vi "Read Frequency.vi"(8 "error in (no error)":errorcluster, 11 "Set Frequency Message in":refnum<class "Set Frequency Message.lvclass">) -> (0 "error out":errorcluster, 2 "Frequency":dbl, 3 "Set Frequency Message out":refnum<class "Set Frequency Message.lvclass">)   [LabVIEW 2011, in "Set Frequency Message.lvclass"]
uses:
  Set Frequency Message.lvclass
  Set Frequency Message.lvclass/Set Frequency Message.ctl
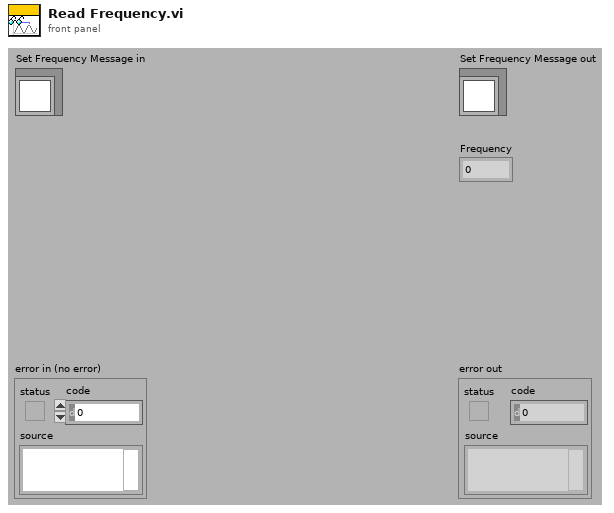
[diagram p1: front panel]
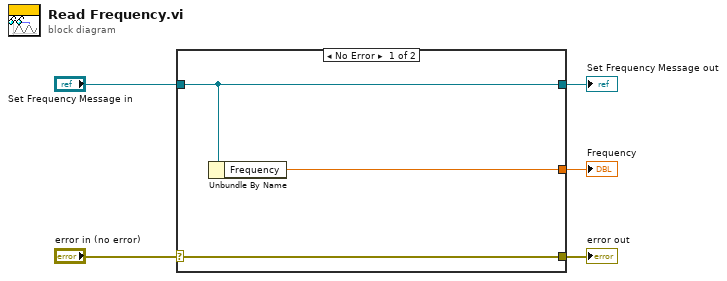
[diagram p0: block diagram]
diagram:
  n1 = case shown="No Error" "error in (no error)" {
    selector: "error in (no error)" -> [w8 w9]
    tunnel: [w8 w9] -> w4
    tunnel: [w7 w10] -> w2
    tunnel: "Set Frequency Message in" -> [w7 w10]
    tunnel: [w6 _] -> w1
    frame No Error {
      n2 = Unbundle By Name(w7) -> ("Frequency"=w6:dbl)
    }
    frame Error {
    }
  }
  "error out" <- w4
  "Set Frequency Message out" <- w2
  "Frequency" <- w1
